vi "Destroy.vi"(8 "Error In":errorcluster, 11 "KnownHosts":refnum<class "KnownHosts.lvclass">) -> (0 "Error Out":errorcluster, 3 "Session":refnum<class "Session.lvclass">)   [LabVIEW 2018, in "Toolkit.lvlib" / "KnownHosts.lvclass"]
uses:
  KnownHosts.lvclass
  Session/Session.lvclass
  KnownHosts.lvclass/KnownHosts.ctl
  Toolkit.lvlib
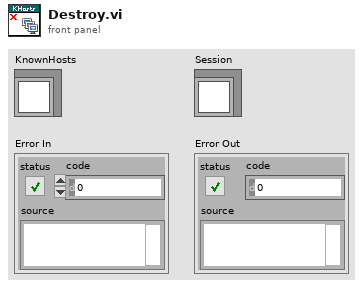
[diagram p1: front panel]
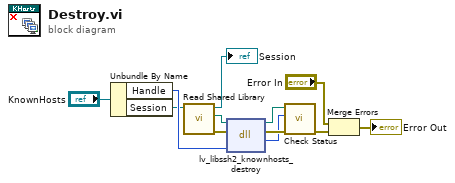
[diagram p0: block diagram]
diagram:
  n1 = Unbundle By Name("KnownHosts") -> ("Handle"=w9:u64, "Session"=w4:refnum<class "Session.lvclass">)
  n2 = call "Read Shared Library.vi"("Session In"=w4) -> ("Erorr Out"=w2:errorcluster, "lv-libssh2 Shared Library"=w3:path, "Session Out"=→"Session":refnum<class "Session.lvclass">)  [unwired: 8 in]
  n3 = dll-call lib="D:/Users/cfield/Code/Field R&D Services/SSH/LV-LIBSSH2/LabVIEW/trunk/src/Toolkit/Support/lv-libssh2.*" fn="lv_libssh2_knownhosts_destroy"(path in=w3, error in=w2, "handle"=w9) -> (path out=w7:path, error out=w8:errorcluster, "status"=w6:i32)  [unwired: 2 in]
  n4 = call "Check Status.vi"("Error In"=w8, "Status"=w6, "lv-libssh2 Shared Library In"=w7) -> ("Error Out"=w5:errorcluster)  [unwired: 7 in, 1 out]
  n5 = Merge Errors("Error In", w5) -> (→"Error Out":errorcluster)
